vi "Drag Stage Position_YCC.vi"() -> ()   [LabVIEW 2014]
uses:
  (Global) Current handle and LaserPower_YCC.vi
panel:
  in  "Move?":bool
  in  "Adjust to  2":bool
  out "Z Current Position (um)":dbl
  in  "Z Move to (um)":dbl=50.0 format="%_6g"
  in  "Y Move to (um)":dbl=50.0 format="%_6f"
  in  "X Move to (um)":dbl=50.0 format="%_6f"
  in  "Darg Mode?":bool=TRUE
  in  "Z Position (um)":dbl=50.0 format="%.4f"
  in  "Move to (50,50,50) ?":bool
  in  "stop":bool
  out "XY Position":cluster{"X":dbl, "Y":dbl}[](graph)
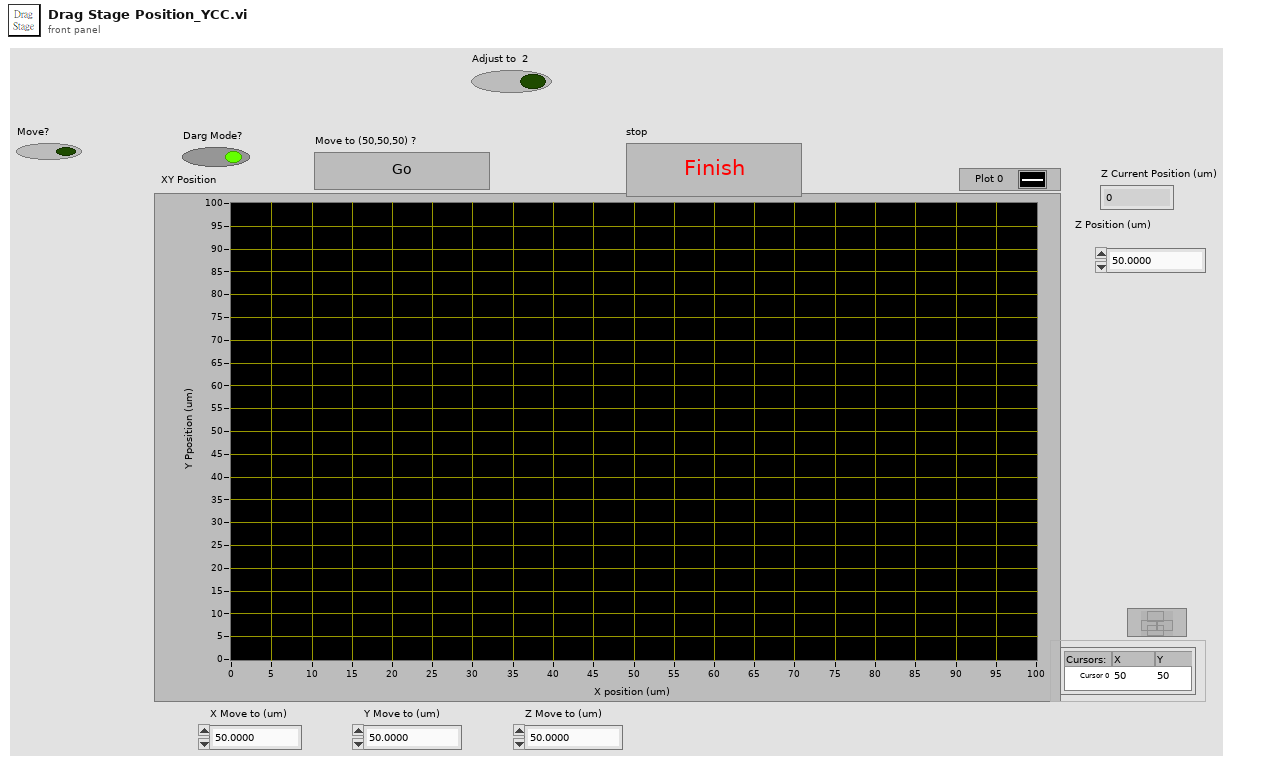
[diagram p1: front panel]
types:
  T1 = cluster{"position (um)":dbl, "position (um)":dbl}
  T2 = cluster{"X Move to (um)":dbl, "Y Move to (um)":dbl}
  T3 = typedef "LVPointDoubleTypeDef.ctl" = cluster{"Cursor X":dbl, "Cursor Y":dbl}
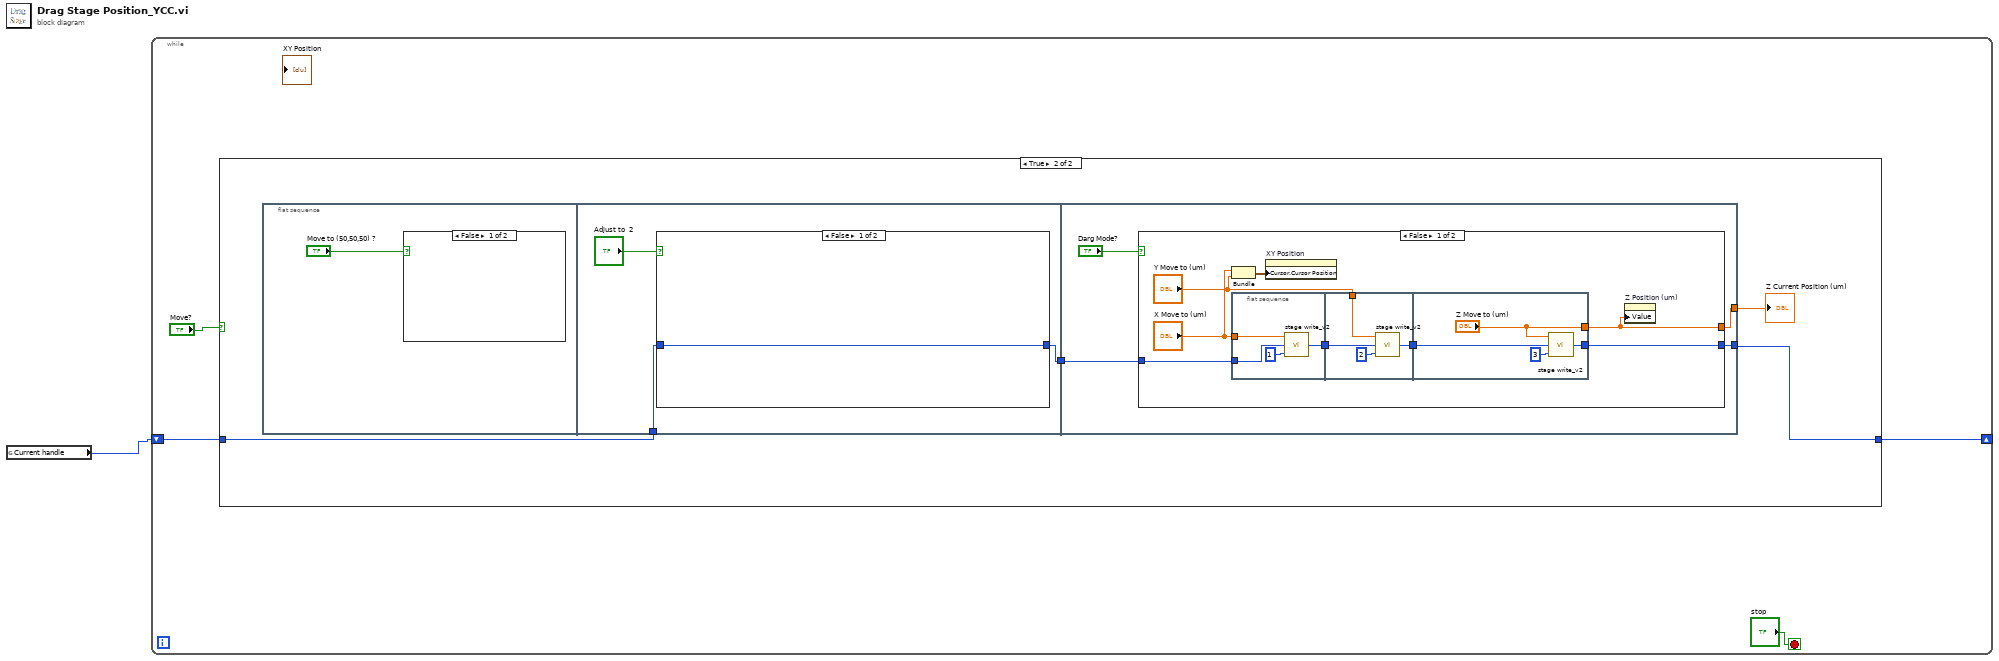
[diagram p0: block diagram]
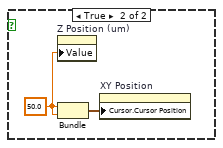
[diagram p3: hidden frame]
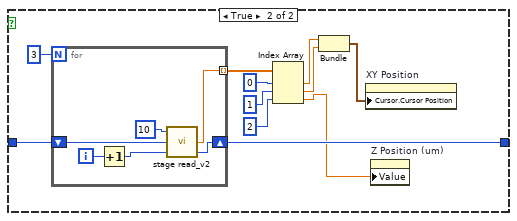
[diagram p4: hidden frame]
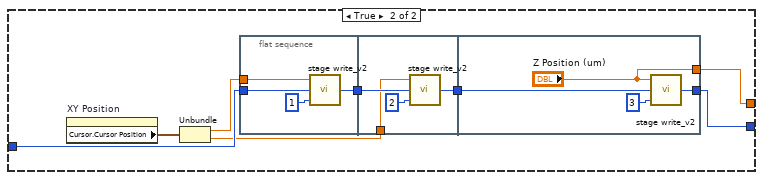
[diagram p5: hidden frame]
diagram:
  n1 = global read "(Global) Current handle and LaserPower_YCC.vi" "Current handle"() -> (w1:i32)
  n2 = while {
    shift-right: [w3] -> _
    shift-left: w1 -> [w4]
    stop <- "stop" stop-if-true
    n3 = case shown="True" "Move?" {
      tunnel: w4 -> [w6 w9]
      tunnel: [w6 w8] -> w3
      frame False {
      }
      frame True {
        n4 = flat-sequence {
          tunnel: w9 -> [w15]
          tunnel: [w14] -> w10
          tunnel: w10 -> [w37]
          tunnel: [w36] -> w8
          tunnel: [w35] -> w7
          frame #0 {
            n5 = case shown="False" "Move to (50,50,50) ?" {
              frame False {
              }
              frame True {
                w12 = 50.0
                n6 = property on="Z Position (um)" class="DigNum (strict)"("Value"=w12) -> ()  [unwired: 2 in, 2 out]
                n7 = Bundle(w12, w12) -> (w13:cluster{dbl, dbl})  [unwired: 1 in]
                n8 = property on="XY Position" class="XYGraph (strict)"("Cursor.Cursor Position"=w13) -> ()  [unwired: 2 in, 2 out]
              }
            }
          }
          frame #1 {
            n9 = case shown="False" "Adjust to  2" {
              tunnel: [w17 w28] -> w14
              tunnel: w15 -> [w17 w27]
              frame False {
              }
              frame True {
                n10 = for {
                  N: 3 -> [_]
                  shift-right: [w29] -> w28
                  shift-left: w27 -> [w31]
                  tunnel: [w30] -> w25 mode=indexing
                  i -> [w34]
                  n11 = Increment(x=w34) -> (x+1=w32:i32)
                  n12 = call "stage read_v2.vi"("Axis"=w32, "Incoming Handle"=w31, "read #"=10) -> ("Outgoing Handle"=w29:i32, "position (um)"=w30:dbl)  [unwired: 1 in]
                }
                n13 = Index Array(array=w25, index #1=0 ("index"), index #2=1 ("index"), index #3=2 ("index")) -> (element #1=w21:dbl, element #2=w20:dbl, element #3=w19:dbl)
                n14 = Bundle("position (um)"=w21, "position (um)"=w20) -> (w18:T1)  [unwired: 1 in]
                n15 = property on="XY Position" class="XYGraph (strict)"("Cursor.Cursor Position"=w18) -> ()  [unwired: 2 in, 2 out]
                n16 = property on="Z Position (um)" class="DigNum (strict)"("Value"=w19) -> ()  [unwired: 2 in, 2 out]
              }
            }
          }
          frame #2 {
            n17 = case shown="False" "Darg Mode?" {
              tunnel: w37 -> [w44 w64]
              tunnel: [w43 w60] -> w36
              tunnel: [w39 w59] -> w35
              frame False {
                n18 = Bundle("X Move to (um)"="X Move to (um)", "Y Move to (um)"="Y Move to (um)") -> (w40:T2)  [unwired: 1 in]
                n19 = flat-sequence {
                  tunnel: w44 -> [w50]
                  tunnel: [w48] -> w46
                  tunnel: "X Move to (um)" -> [w47]
                  tunnel: w46 -> [w53]
                  tunnel: "Y Move to (um)" -> [w52]
                  tunnel: [w51] -> w45
                  tunnel: [w56] -> w43
                  tunnel: w45 -> [w57]
                  tunnel: ["Z Move to (um)"] -> w39
                  frame #0 {
                    n20 = call "stage write_v2.vi"("axis"=u32 1, "Incoming Handle"=w50, "position"=w47) -> ("out handle"=w48:i32)  [unwired: 2 in]
                  }
                  frame #1 {
                    n21 = call "stage write_v2.vi"("axis"=u32 2, "Incoming Handle"=w53, "position"=w52) -> ("out handle"=w51:i32)  [unwired: 2 in]
                  }
                  frame #2 {
                    n22 = call "stage write_v2.vi"("axis"=u32 3, "Incoming Handle"=w57, "position"="Z Move to (um)") -> ("out handle"=w56:i32)  [unwired: 2 in]
                  }
                }
                n23 = property on="XY Position" class="XYGraph (strict)"("Cursor.Cursor Position"=w40) -> ()  [unwired: 2 in, 2 out]
                n24 = property on="Z Position (um)" class="DigNum (strict)"("Value"=w39) -> ()  [unwired: 2 in, 2 out]
              }
              frame True {
                n25 = property on="XY Position" class="XYGraph (strict)"() -> ("Cursor.Cursor Position"=w63:T3)  [unwired: 2 in, 2 out]
                n26 = Unbundle(w63) -> ("Cursor X"=w62:dbl, "Cursor Y"=w61:dbl)
                n27 = flat-sequence {
                  tunnel: w64 -> [w70]
                  tunnel: [w68] -> w66
                  tunnel: w62 -> [w67]
                  tunnel: w66 -> [w73]
                  tunnel: w61 -> [w72]
                  tunnel: [w71] -> w65
                  tunnel: w65 -> [w77]
                  tunnel: [w76] -> w60
                  tunnel: ["Z Position (um)"] -> w59
                  frame #0 {
                    n28 = call "stage write_v2.vi"("axis"=u32 1, "Incoming Handle"=w70, "position"=w67) -> ("out handle"=w68:i32)  [unwired: 2 in]
                  }
                  frame #1 {
                    n29 = call "stage write_v2.vi"("axis"=u32 2, "Incoming Handle"=w73, "position"=w72) -> ("out handle"=w71:i32)  [unwired: 2 in]
                  }
                  frame #2 {
                    n30 = call "stage write_v2.vi"("axis"=u32 3, "Incoming Handle"=w77, "position"="Z Position (um)") -> ("out handle"=w76:i32)  [unwired: 2 in]
                  }
                }
              }
            }
          }
        }
        "Z Current Position (um)" <- w7
      }
    }
  }
